vi "Numeric Case Structure.vi"() -> ()   [LabVIEW 2023]
panel:
  in  "Fahrenheit?":i32
  in  "stop":bool
  out "Temperature Output":dbl(slide) scale=0.0..2000.0
  in  "Celsius Input":dbl(slide) scale=0.0..1000.0
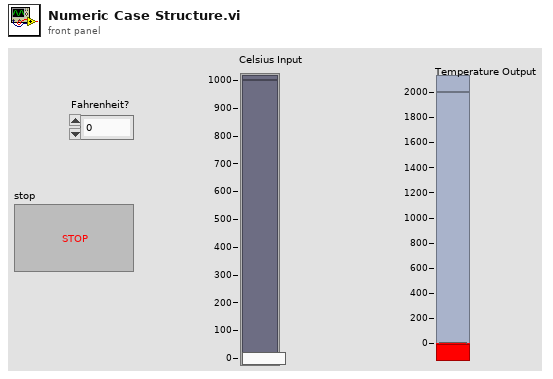
[diagram p1: front panel]
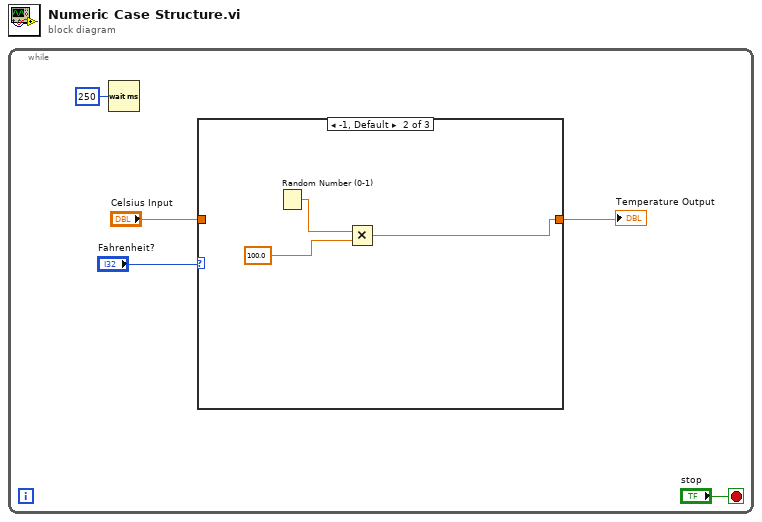
[diagram p0: block diagram]
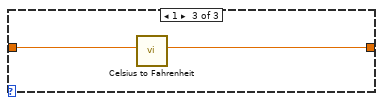
[diagram p3: hidden frame]
diagram:
  n1 = while {
    stop <- "stop" stop-if-true
    n2 = Wait (ms)(milliseconds to wait=u32 250) -> ()  [unwired: 1 out]
    n3 = case shown="-1, Default" "Fahrenheit?" {
      tunnel: "Celsius Input" -> [w6 _ w11]
      tunnel: [w6 w7 w10] -> w2
      frame 0 {
      }
      frame -1, Default {
        n4 = Random Number (0-1)() -> (number: 0 to 1=w9:dbl)
        n5 = Multiply(x=w9, y=100.0) -> (x*y=w7:dbl)
      }
      frame 1 {
        n6 = call "Celsius to Fahrenheit.vi"("Celsius"=w11) -> ("Fahrenheit"=w10:dbl)  [unwired: 10 in]
      }
    }
    "Temperature Output" <- w2
  }
